vi "Save HW as XML.vi"(8 "error in (no error)":errorcluster, 10 "Path":path, 11 "Hardware Settings.lvclass":refnum<class "Hardware Settings.lvclass">) -> (0 "error out":errorcluster)   [LabVIEW 2017, in "Hardware Settings.lvclass"]
uses:
  Hardware Settings.lvclass
  <vilib>/Utility/xml.llb/Write to XML File(string).vi
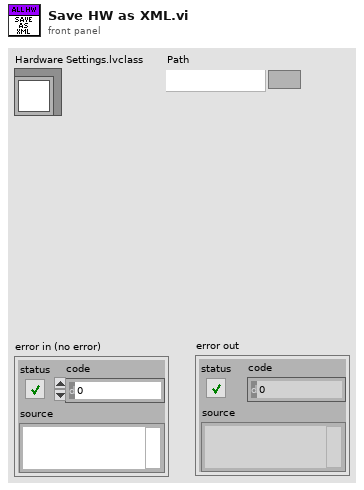
[diagram p1: front panel]
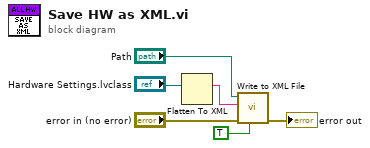
[diagram p0: block diagram]
diagram:
  n1 = Flatten To XML(anything="Hardware Settings.lvclass") -> (xml string=w4:string)
  n2 = call-poly <vilib>:"Write to XML File.vi"("Standalone? (T)"=TRUE, "error in (no error)"="error in (no error)", "XML Input"=w4, "XML File Path"="Path") -> ("error out"=→"error out":errorcluster)  [unwired: 5 in, 2 out]
